vi "VD-setSettingseasy.vi"(8 "error in (no error)":errorcluster, 10 "settings":T1 {"sampleSize" items=["101"=101, "201"=201, "401"=401, "601"=601, "801"=801, "1001"=1001]; "Stop [hz]" format="%.0p"; "Start [hz]" format="%.0p"}, 11 "VD-LV-LiteVNA in":refnum<class "VD-LV-LiteVNA.lvclass">) -> (0 "error out":errorcluster, 3 "VD-LV-LiteVNA out":refnum<class "VD-LV-LiteVNA.lvclass">)   [LabVIEW 2020, in "VD-LV-LiteVNA.lvclass"]
uses:
  VD-LV-LiteVNA.lvclass
  VD-settingsEasy.ctl
  VD-sampleSize.ctl
  VD-settings.ctl
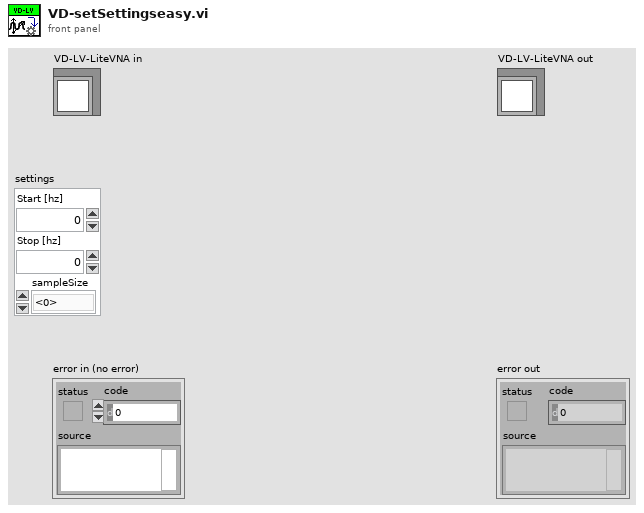
[diagram p1: front panel]
types:
  T1 = typedef "VD-LV-LiteVNA.lvclass/VD-settingsEasy.ctl" = cluster{"Start [hz]":u64, "Stop [hz]":u64, "sampleSize":T2}
  T2 = typedef "VD-LV-LiteVNA.lvclass/VD-sampleSize.ctl" = u16
  T3 = typedef "VD-LV-LiteVNA.lvclass/VD-settings.ctl" = cluster{"Start [Hz]":u64, "Span [Hz]":u64, "Number of points #":u16, "Sample Average #":u16}
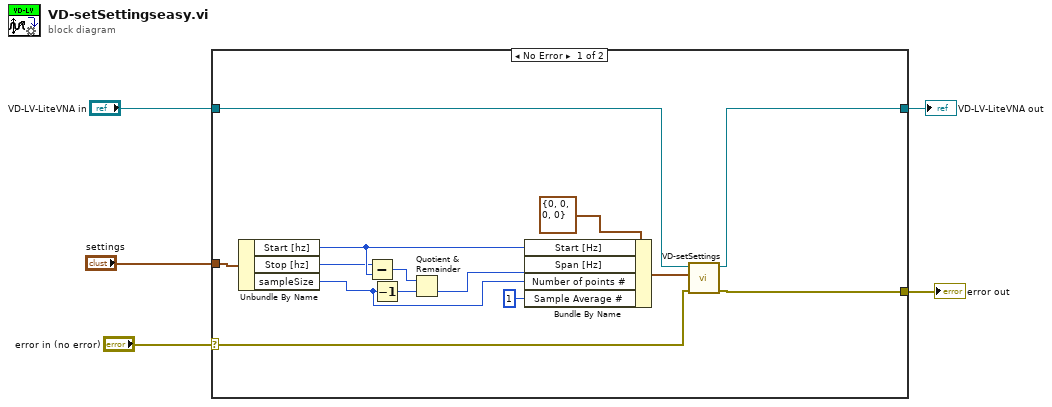
[diagram p0: block diagram]
diagram:
  n1 = case shown="No Error" "error in (no error)" {
    selector: "error in (no error)" -> [w9 w21]
    tunnel: [w8 w21] -> w4
    tunnel: [w7 w20] -> w2
    tunnel: "VD-LV-LiteVNA in" -> [w19 w20]
    tunnel: "settings" -> [w16 _]
    frame No Error {
      n2 = Unbundle By Name(w16) -> ("Start [hz]"=w15:u64, "Stop [hz]"=w14:u64, "sampleSize"=w11:T2)
      n3 = Subtract(x=w14, y=w15) -> (x-y=w13:u64)
      n4 = Decrement(x=w11) -> (x-1=w6:T2)
      n5 = Quotient & Remainder(x=w13, y=w6) -> (floor(x/y)=w12:u64)  [unwired: 1 out]
      n6 = Bundle By Name(cluster=T3 {"Start [Hz]"=0, "Span [Hz]"=0, "Number of points #"=0, "Sample Average #"=0} ("Settings"), "Start [Hz]"=w15, "Span [Hz]"=w12, "Number of points #"=w11, "Sample Average #"=u16 1) -> (w17:T3)
      n7 = call "VD-setSettings.vi"("error in (no error)"=w9, "Settings"=w17, "VD-LV-LiteVNA in"=w19) -> ("error out"=w8:errorcluster, "VD-LV-LiteVNA out"=w7:refnum<class "VD-LV-LiteVNA.lvclass">)  [unwired: 7 in]
    }
    frame Error {
    }
  }
  "error out" <- w4
  "VD-LV-LiteVNA out" <- w2
